vi "Stop Core.vi"(10 "final error code":i32, 11 "UI Base in":refnum<class "UI Base.lvclass">) -> (3 "UI Base out":refnum<class "UI Base.lvclass">)   [LabVIEW 2023, in "UI Base.lvlib" / "UI Base.lvclass"]
doc: "(<B>Filename</B>: Actor Framework.lvlib:Actor.lvclass:Stop Core.vi)\n\nDefines what the actor does before it stops. Use the <B>final error code</B> input to determine whether the actor shut down in response to an error.\n\nBy default, this method passes the Stop message along to all auto-stop nested actors. A descendant class may override this method to define additional behavior, such as shutting down any processes the actor initiated in its override of the Actor Core method."
uses:
  UI Base.lvclass
  UI Base.lvclass/UI Base.ctl
  <vilib>/ActorFramework/Actor/Actor.lvclass
  Interfaces/Incoming Model Base Interface Messages/UI Closed Msg/UI Closed Msg.lvclass
  C:/Program Files/National Instruments/LabVIEW 2023/vi.lib/ActorFramework/Actor/Actor.lvclass
  C:/Users/bhaghyaraj/Trainings/NI Actor Frameowork/SDLC/UI Base/UI Base/UI Base.lvclass
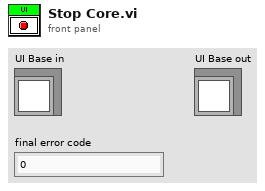
[diagram p1: front panel]
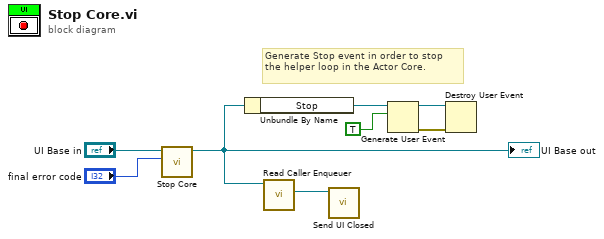
[diagram p0: block diagram]
diagram:
  # "Generate Stop event in order to stop the helper loop in the Actor Core."
  n1 = call-parent "Stop Core.vi"("final error code"="final error code", "Actor in"="UI Base in") -> ("Actor out"=w2:refnum<class "UI Base.lvclass">)  [unwired: 9 in]
  "UI Base out" <- w2
  n2 = Unbundle By Name(w2) -> ("Stop"=w4:refnum<user-event>)
  n3 = call <vilib>:"Read Caller Enqueuer.vi"("Actor"=w2) -> ("Caller Enqueuer"=w1:refnum<class "Message Enqueuer.lvclass">)  [unwired: 10 in]
  n4 = call "Send UI Closed.vi"("Message Enqueuer"=w1) -> ()  [unwired: 9 in, 2 out]
  n5 = Generate User Event(user event=w4, event data cluster=TRUE ("event data")) -> (user event out=w6:refnum<user-event>, error out=w5:errorcluster)  [unwired: 2 in]
  n6 = Destroy User Event(user event=w6, error in=w5) -> ()  [unwired: 1 out]
